vi "CFG Handle P20 ATP Sequence Paths.vi"(0 "Path":path, 1 "Section":string, 11 "Error In (no error)":errorcluster) -> (4 "ATP Relative Path":path, 8 "Start Path":path, 15 "error out":errorcluster)   [LabVIEW 2017]
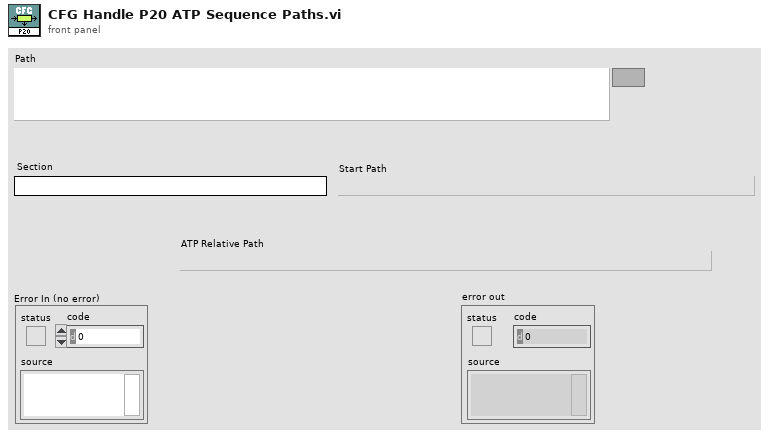
[diagram p1: front panel]
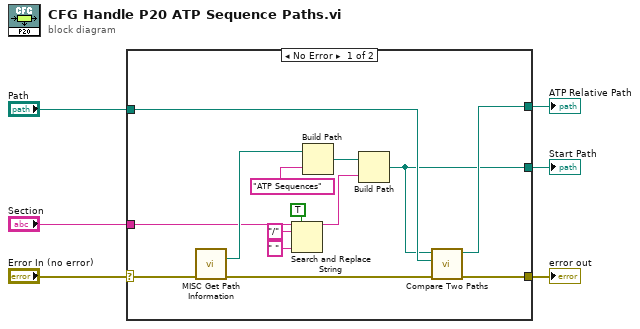
[diagram p0: block diagram]
diagram:
  n1 = case shown="No Error" "Error In (no error)" {
    selector: "Error In (no error)" -> [w16 w21]
    tunnel: "Path" -> [w14 _]
    tunnel: "Section" -> [w11 _]
    tunnel: [w18 w21] -> w4
    tunnel: [w15 _] -> w2
    tunnel: [w7 _] -> w1
    frame No Error {
      n2 = call "MISC Get Path Information.vi"("Error In (no error)"=w16) -> ("Application Directory"=w13:path, "Error Out"=w19:errorcluster)  [unwired: 13 out]
      n3 = Search and Replace String(replace all?=TRUE ("replace all? (F)"), input string=w11, search string="/", replace string=" " ("replace string (\"\")")) -> (result string=w8:string)  [unwired: 1 in, 6 out]
      n4 = Build Path(base path=w13, name or relative path="ATP Sequences") -> (appended path=w20:path)
      n5 = Build Path(base path=w20, name or relative path=w8) -> (appended path=w7:path)
      n6 = call <vilib>:"Compare Two Paths.vi"("error in (no error)"=w19, "Path 2"=w14, "Path 1"=w7) -> ("error out"=w18:errorcluster, "Relative Path from 1 to 2"=w15:path)  [unwired: 7 out]
    }
    frame Error {
    }
  }
  "error out" <- w4
  "ATP Relative Path" <- w2
  "Start Path" <- w1
